vi "getViGeneralInfo.vi"(8 "error in (no error)":errorcluster, 11 "VI in":refnum<vi>) -> (0 "error out":errorcluster, 2 "VI General Info":T2, 3 "VI out":refnum<vi>)   [LabVIEW 2017, in "vi_tools.lvlib"]
doc: "Returns the general information for the specified VI reference."
uses:
  vi_tools.lvlib
  connectorPanePatterns.ctl
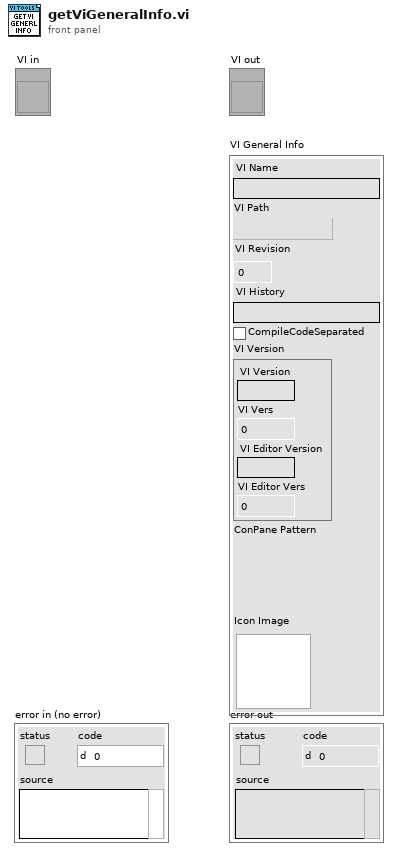
[diagram p1: front panel]
types:
  T1 = typedef "vi_tools.lvlib/connectorPanePatterns.ctl" = i32
  T2 = cluster{"VI Name":string, "VI Path":path, "VI Revision":u32, "VI History":string, "CompileCodeSeparated":bool, "VI Version":cluster{"VI Version":string, "VI Vers":u32, "VI Editor Version":string, "VI Editor Vers":u32}, "ConPane Pattern":T1, "Icon Image":picture}
  T3 = cluster{"GetVIVers":string, "VI Path":u32, "Get VI Editor Version":string, "Vers Num":u32}
  T4 = typedef "imagedata.ctl" = cluster{"image type":i32, "image depth":i32, "image":u8[], "mask":u8[], "colors":u32[], "Rectangle":cluster{"left":i16, "top":i16, "right":i16, "bottom":i16}}
  T5 = cluster{"Name":string, "Path":path, "Hist.Revision":u32, "Hist.Text":string, bool, "Version":cluster{"GetVIVers":string, "VI Path":u32, "Get VI Editor Version":string, "Vers Num":u32}, "Connector Pane Patterns":T1, "new picture":picture}
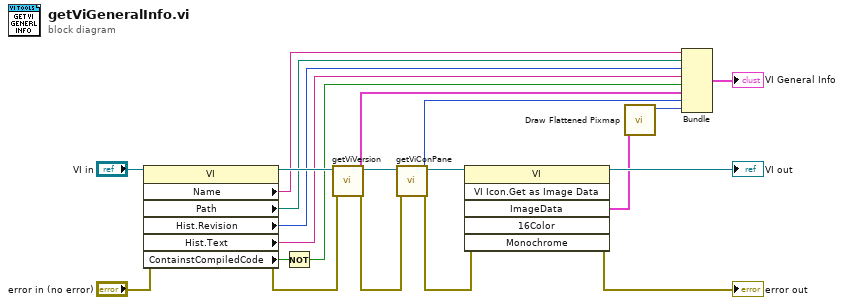
[diagram p0: block diagram]
diagram:
  n1 = property class="VI"(reference="VI in", error in="error in (no error)") -> (reference out=w19:refnum<vi>, error out=w17:errorcluster, "Name"=w16:string, "Path"=w15:path, "Hist.Revision"=w14:u32, "Hist.Text"=w13:string, "ContainstCompiledCode"=w10:bool)
  n2 = Not(x=w10) -> (.not. x?=w9:bool)
  n3 = call "getViVersion.vi"("error in (no error)"=w17, "VI in"=w19) -> ("error out"=w6:errorcluster, "Version"=w11:T3, "VI out"=w18:refnum<vi>)  [unwired: 7 in]
  n4 = call "getViConPane.vi"("error in (no error)"=w6, "VI in"=w18) -> ("error out"=w1:errorcluster, "Connector Pane Patterns"=w2:T1, "VI out"=w7:refnum<vi>)  [unwired: 7 in]
  n5 = invoke class="VI" method="VI Icon.Get as Image Data"(reference=w7, error in=w1) -> (reference out=→"VI out":refnum<vi>, error out=→"error out":errorcluster, "ImageData"=w4:T4)  [unwired: 4 in, 3 out]
  n6 = call <vilib>:"Draw Flattened Pixmap.vi"("image data"=w4) -> ("new picture"=w3:picture)  [unwired: 8 in]
  n7 = Bundle("Name"=w16, "Path"=w15, "Hist.Revision"=w14, "Hist.Text"=w13, w9, "Version"=w11, "Connector Pane Patterns"=w2, "new picture"=w3) -> (→"VI General Info":T5)  [unwired: 1 in]
